vi "Append Path to Root if Relative - Scalar__ogtk.vi"(1 "Absolute or Relative Path":path, 2 "Root Path":path) -> (0 "Absolute or Appended Path":path)   [LabVIEW 2018]
doc: "Ouputs \"Absolute or Relative Path\". If \"Absolute or Relative Path\" is relative it is appended to \"Root Path\". If \"Absolute or Relative Path\" is absolute it is passed straight through."
panel:
  # "Append Path to Root if Relative.vi\n\nAppends a path to the Root Path if the path is relative, or outputs the path if it is absolute.\n\nPlease visit http://www.OpenG.org to learn about the\nOpen Source LabVIEW software movement.\n\nNOTICE -- YOU MUST LEAVE THIS NOTICE IN PLACE.  PER THE TERMS OF THE LICENSE BELOW, YOU MAY SUBLICENSE THIS SOFTWARE \nIN ANY WAY THAT DOES NOT CONFLICT WITH THIS LICENSE.\n\n### BSD License (http://www.opensource.org/licenses/bsd-license.php) Begin ###\n \nCopyright (c) 2002-2006, Jim Kring <jim@jimkring.com>\nCopyright (c) 2010, Jonathon Green <jg@jgcode.net>\n\nAll rights reserved.\n\nRedistribution and use in source and binary forms, with or without modification, are permitted provided that the following conditions are met:\n\n    * Redistributions of source code must retain the above copyright notice, this list of conditions and the following disclaimer.\n    * Redistributions in binary form must reproduce the above copyright notice, this list of conditions and the following disclaimer in the \n       documentation and/or other materials provided with the distribution.\n    * Neither the name of SciWare, James Kring, Inc., nor the names of its contributors may be used to endorse or promote products derived \n       from this software without specific prior written permission.\n\nTHIS SOFTWARE IS PROVIDED BY THE COPYRIGHT HOLDERS AND CONTRIBUTORS \"AS IS\" AND ANY EXPRESS OR IMPLIED WARRANTIES, \nINCLUDING, BUT NOT LIMITED TO, THE IMPLIED WARRANTIES OF MERCHANTABILITY AND FITNESS FOR A PARTICULAR PURPOSE ARE \nDISCLAIMED. IN NO EVENT SHALL THE COPYRIGHT OWNER OR CONTRIBUTORS BE LIABLE FOR ANY DIRECT, INDIRECT, INCIDENTAL,\n SPECIAL, EXEMPLARY, OR CONSEQUENTIAL DAMAGES (INCLUDING, BUT NOT LIMITED TO, PROCUREMENT OF SUBSTITUTE GOODS OR \nSERVICES; LOSS OF USE, DATA, OR PROFITS; OR BUSINESS INTERRUPTION) HOWEVER CAUSED AND ON ANY THEORY OF LIABILITY, \nWHETHER IN CONTRACT, STRICT LIABILITY, OR TORT (INCLUDING NEGLIGENCE OR OTHERWISE) ARISING IN ANY WAY OUT OF THE USE \nOF THIS SOFTWARE, EVEN IF ADVISED OF THE POSSIBILITY OF SUCH DAMAGE.\n\n### BSD License End ###"
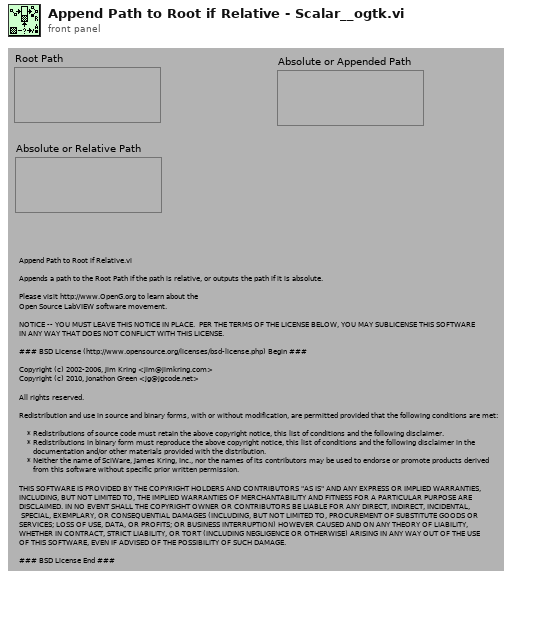
[diagram p1: front panel]
types:
  T1 = enum16{"Absolute path", "Relative path", "Not-a-path"}
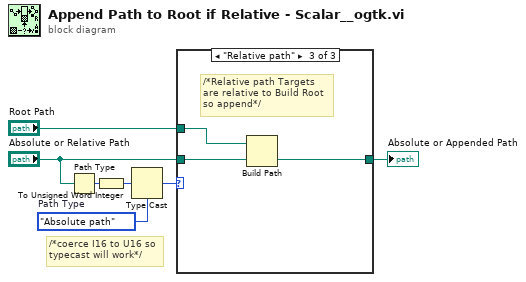
[diagram p0: block diagram]
diagram:
  w2 = T1."Absolute path"  # Path Type
  # "/*coerce I16 to U16 so typecast will work*/"
  n1 = Path Type(1:"Absolute or Relative Path") -> (0:w1:i16)
  n2 = To Unsigned Word Integer(number=w1) -> (unsigned 16bit integer=w3:u16)
  n3 = Type Cast(type=w2, x=w3) -> (*(type *) &x=w4:T1)
  n4 = case shown="\"Relative path\"" w4 {
    tunnel: "Absolute or Relative Path" -> [w8 w9 w11]
    tunnel: [w8 w9 w10] -> w6
    tunnel: "Root Path" -> [_ _ w12]
    frame "Absolute path" {
      # "/*Pass absolute paths through*/"
    }
    frame "Not-a-path" {
      # "/*Not-a-path is an error*/"
    }
    frame "Relative path" {
      # "/*Relative path Targets are relative to Build Root so append*/"
      n5 = Build Path(base path=w12, name or relative path=w11) -> (appended path=w10:path)
    }
  }
  "Absolute or Appended Path" <- w6
